vi "Retrieve All Characters.vi"(8 "error in (no error)":errorcluster, 11 "xwpfReader in":refnum<class "xwpfReader.lvclass">) -> (0 "error out":errorcluster, 2 "All Characters":string, 3 "xwpfReader out":refnum<class "xwpfReader.lvclass">)   [LabVIEW 2017, in "LabVIEW NPOI.lvlib" / "xwpfReader.lvclass"]
doc: "Retrieves all the text from the document.\n\nThis VI uses an XWPFTextExtractor to extract the textual content of the document."
uses:
  xwpfReader.lvclass
  xwpfReader.lvclass/xwpfReader.ctl
  C:/Users/Neo/Desktop/Dev_Tools_BR/LabVIEW_NPOI/lib/NPOI 2.1.1/NPOI.OOXML.dll
  lib/NPOI 2.1.1/NPOI.OOXML.dll
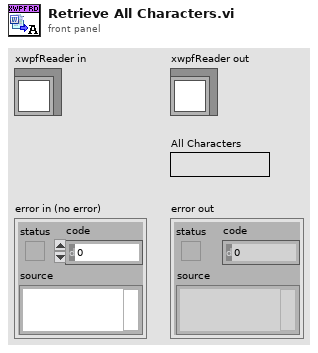
[diagram p1: front panel]
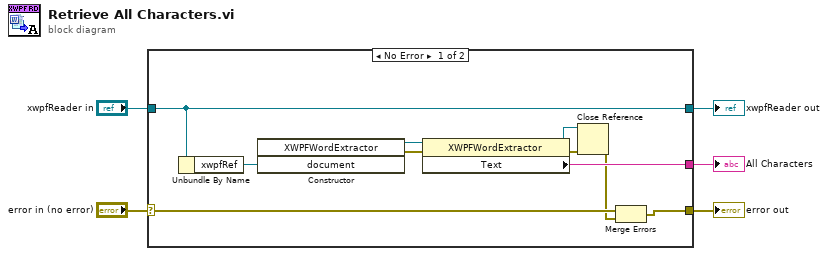
[diagram p0: block diagram]
diagram:
  n1 = case shown="No Error" "error in (no error)" {
    selector: "error in (no error)" -> [w15 w17]
    tunnel: [w7 w17] -> w4
    tunnel: [w14 w16] -> w2
    tunnel: "xwpfReader in" -> [w14 w16]
    tunnel: [w10 _] -> w1
    frame No Error {
      n2 = Unbundle By Name(w14) -> ("xwpfRef"=w13:refnum<k24>)
      n3 = constructor class="XWPFWordExtractor"("document"=w13) -> (reference out=w11:refnum<k24>, error out=w12:errorcluster)  [unwired: 3 in, 2 out]
      n4 = property class="XWPFWordExtractor"(reference=w11, error in=w12) -> (reference out=w9:refnum<k24>, error out=w8:errorcluster, "Text"=w10:string)
      n5 = Close Reference(reference=w9, error in (no error)=w8) -> (error out=w6:errorcluster)
      n6 = Merge Errors(w15, w6) -> (w7:errorcluster)
    }
    frame Error {
    }
  }
  "error out" <- w4
  "xwpfReader out" <- w2
  "All Characters" <- w1
